vi "channel settings to type and function support.vi"(8 "error in":errorcluster, 11 "FixedChannelTBModuleDecideFeatures in":refnum<class "FixedChannelTBModuleDecideFeatures.lvclass">) -> (0 "error out":errorcluster, 3 "FixedChannelTBModuleDecideFeatures out":refnum<class "FixedChannelTBModuleDecideFeatures.lvclass">)   [LabVIEW 2013, in "FixedChannelTBModuleDecideFeatures.lvclass"]
uses:
  FixedChannelTBModuleDecideFeatures.lvclass
  <vilib>/NI/Tag Bus/tag/Data Type.ctl
  FixedChannelTBModuleDecideFeatures.lvclass/FixedChannelTBModuleDecideFeatures.ctl
  <vilib>/NI/Tag Bus/tag/tag descriptor.lvclass
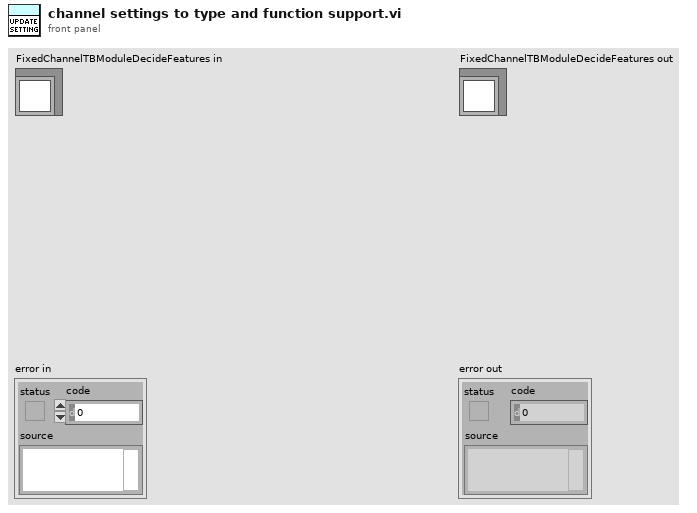
[diagram p1: front panel]
types:
  T1 = typedef "tag bus.lvlib/tag descriptor.lvclass/Data Type.ctl" = enum16{"Double", "Single", "I64", "I32", "I16", "I8", "U64", "U32", "U16", "U8", "Boolean", "String", "Array of Double", "Array of Single", "Array of I64", "Array of I32", "Array of I16", "Array of I8", "Array of U64", "Array of U32", "Array of U16", "Array of U8", "Array of Boolean", "Array of String"}
  T2 = typedef "FixedChannelTBModuleDecideFeatures.lvclass/channel configuration.ctl" = cluster{"Name":string, "channel classification":T3, "data type":T1}
  T3 = typedef "TBM channel.lvclass/channel classification.ctl" = enum16{"input data", "output data", "processing parameter", "processing result"}
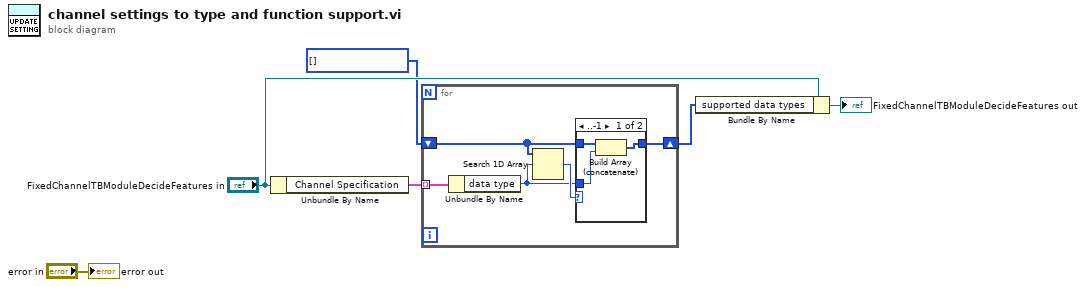
[diagram p0: block diagram]
diagram:
  w2 = T1[] [] items=["Double", "Single", "I64", "I32", "I16", "I8", "U64", "U32", "U16", "U8", "Boolean", "String", "Array of Double", "Array of Single", "Array of I64", "Array of I32", "Array of I16", "Array of I8", "Array of U64", "Array of U32", "Array of U16", "Array of U8", "Array of Boolean", "Array of String"] ("supported data types")
  n1 = Unbundle By Name("FixedChannelTBModuleDecideFeatures in") -> ("Channel Specification"=w3:T2[])
  n2 = for {
    tunnel: w3 -> [w11] mode=indexing
    shift-right: [w9] -> w1
    shift-left: w2 -> [w8]
    n3 = Unbundle By Name(w11) -> ("data type"=w7:T1)
    n4 = Search 1D Array(1D array=w8, element=w7) -> (index of element=w10:i32)  [unwired: 1 in]
    n5 = case shown="..-1" w10 {
      tunnel: [w12 w15] -> w9
      tunnel: w8 -> [w14 w15]
      tunnel: w7 -> [w13 _]
      frame ..-1 {
        n6 = Build Array (concatenate)(w14, w13) -> (w12:T1[])
      }
      frame 0.. {
      }
    }
  }
  n7 = Bundle By Name(cluster="FixedChannelTBModuleDecideFeatures in", "supported data types"=w1) -> (→"FixedChannelTBModuleDecideFeatures out":refnum<class "FixedChannelTBModuleDecideFeatures.lvclass">)
  "error out" <- "error in"
